vi "DAQ 1SDI v6.1.vi"() -> ()   [LabVIEW 2013]
uses:
  Strict Type Defs/type_meas_enum.ctl
  <instrlib>/niScope/Controls/niScope vertical coupling.ctl
panel:
  in  "stop":bool
  out "Loop count":i32=4690
  in  "Monitors":T1(tab)
  out "covariance HD 1 & 2":dbl(graph)=0.19831028169384832
  out "Conditional variance HD 1|2":dbl(graph)=1.0142124161365378
  out "Conditional variance HD 1|3":dbl(graph)=0.6065160666682574
  out "Conditional variance HD 2|3":dbl(graph)=0.5661489724627885
  out "covariance HD 1 & 3":dbl(graph)=-0.6559385878875881
  out "covariance HD 2 & 3":dbl(graph)=-0.6106758756892631
  in  "mode 2 polarity":bool
  out "Var(x1-x2/sqrt(2)-x3(sqrt(2))":dbl(graph)=0.19831028169384832
  out "Var(x2-x1/sqrt(2)-x3/sqrt(2))":dbl(graph)=-0.6559385878875881
  out "Var(x3-x1/sqrt(2)-x2/sqrt(2))":dbl(graph)=-0.6106758756892631
  in  "mode 3 polarity":bool
  in  "Settings":enum32{"Settings and Record", "Under the hood"}(tab)=enum."Under the hood"
  in  "Delay timing (ms)":u32(knob)=43 scale=0.0..250.0
  in  "Number of monitor samples":i32=10000 format="%.0p"
  in  "File location":path=path "C:/ni-rt/LabVIEW Data/July1/35dB109"
  in  "Type of measurement":T2=enum."electronic"
  in  "File root name":string="Real"
  in  "Number of samples save":i32=2000000 format="%.0p"
  in  "reset sn":bool
  in  "Shot noise start":bool
  in  "Additional text":string="OPA 1 optical power set to 15mV on HD A.\nOPA 2 optical power set to 15mV on HD B.\nLocal oscillator is set to 5V on HD.\nParametric gain set to 15 for OPA 1.\nParametric gain set to 15 for OPA 2.\nVertical range set to 0.5V for both channels.\nSample rate set to 14MS/s.\nMax input freq set to7MHz.\nVisibility between OPA 1 & OPA 2 = 99.6\nVisibility between OPA 1 & L.O.B = 98.9\nVisibility between OPA 1 & L.O. A = 98.9\nBoth squeezers expected to produce -7dB/11dB.\nLoss on EPR B =55.33% (3.5dB) \n"
  in  "Record":bool
  in  "Number of Files":i32=2
  out "File count":i32=1
  in  "Run":string="9"
  out "Cluster":T3={"Actual samples acquired ch 1"=120000, "Actual samples acquired ch 0"=120000, "Actual samples acquired ch 2"=120000}
  in  "Channel Parms":T5={"Input impedance (Ohms)"=2, "Maximum input frequency (Hz)"=7.0, "vertical coupling"=1, "Probe attenuation"=1.0, "Vertical range (V)"=1.0, "Vertical offset"=0.0, "channel enabled"=TRUE} {"Input impedance (Ohms)" items=["1 mega ohm"=0, "50 ohms"=2]; "Maximum input frequency (Hz)" format="%#_6p"; "vertical coupling" items=["AC", "DC", "Ground"]}
  in  "IIR filter specifications":T6={"Topology"=enum."Butterworth", "Type"=enum."Bandpass", "Order"=6, "Lower Fc"=2900000.0, "Upper Fc"=3100000.0, "PB Ripple"=1.0, "SB Attenuation"=60.0} {"PB Ripple" format="%0.2f"; "SB Attenuation" format="%0.2f"; "Lower Fc" format="%0.2p"; "Upper Fc" format="%0.2p"}
  out "error out":errorcluster caption="error out final"
  in  "max time (s)":dbl=10.0 caption="Time to run (s)"
  in  "Reference position":dbl(slide)=50.0 scale=0.0..100.0
  in  "Minimum sample rate (S/s)":dbl=14000000.0 format="%#_6p"
  out "Video bandwidth (Hz)":dbl=7.0
  in  "DAQ Cards":T7={"DAQ Card 1"="Dev2", "DAQ Card 2"="Dev3"}
  # "+1"
  # "-1"
  # "+1"
  # "-1"
  # "Variance won't be displayed until shot noise is taken"
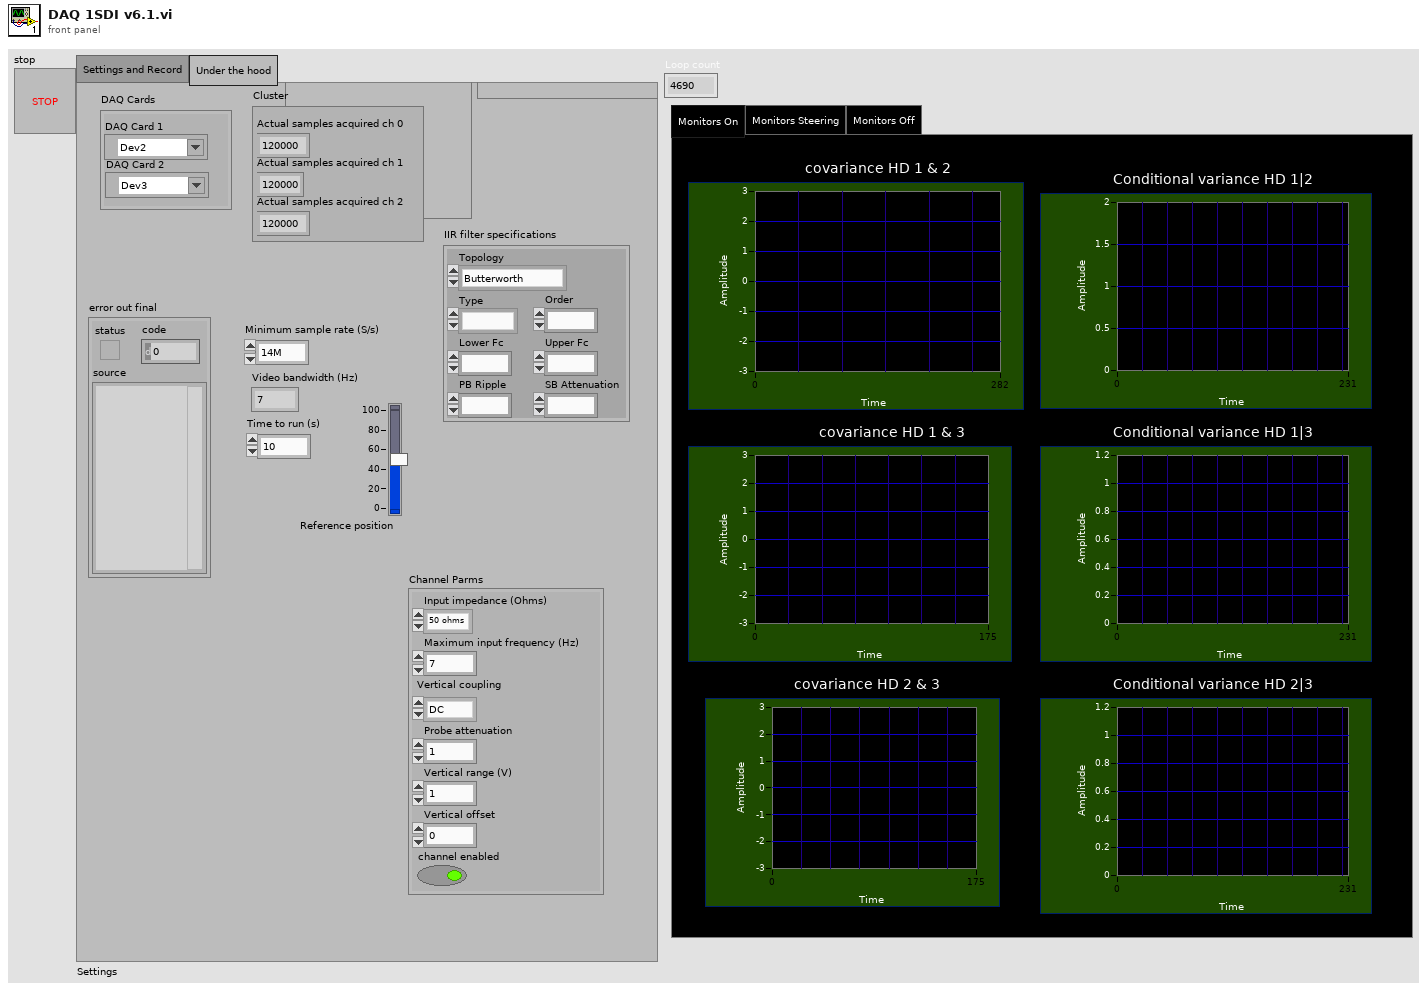
[diagram p1: front panel]
types:
  T1 = enum32{"Monitors On", "Monitors Steering", "Monitors Off"}
  T2 = typedef "type_meas_enum.ctl" = enum16{"shot", "x", "p", "electronic"}
  T3 = cluster{"Actual samples acquired ch 1":i32, "Actual samples acquired ch 0":i32, "Actual samples acquired ch 2":i32}
  T4 = typedef "niScope vertical coupling.ctl" = i32
  T5 = cluster{"Input impedance (Ohms)":u32, "Maximum input frequency (Hz)":dbl, "vertical coupling":T4, "Probe attenuation":dbl, "Vertical range (V)":dbl, "Vertical offset":dbl, "channel enabled":bool}
  T6 = cluster{"Topology":enum16{"Off", "Butterworth", "Chebyshev", "Inverse Chebyshev", "Elliptic", "Bessel"}, "Type":enum16{"Lowpass", "Highpass", "Bandpass", "Bandstop"}, "Order":i32, "Lower Fc":dbl, "Upper Fc":dbl, "PB Ripple":dbl, "SB Attenuation":dbl}
  T7 = cluster{"DAQ Card 1":refnum<k15>, "DAQ Card 2":refnum<k15>}
  T8 = cluster{"instrument handle":refnum<k15>, "instrument handle":refnum<k15>}
  T9 = cluster{"instrument handle out 0":refnum<k15>, "instrument handle out 1":refnum<k15>}
  T10 = cluster{"actualSamples":i32, "actualSamples":i32, "actualSamples":i32}
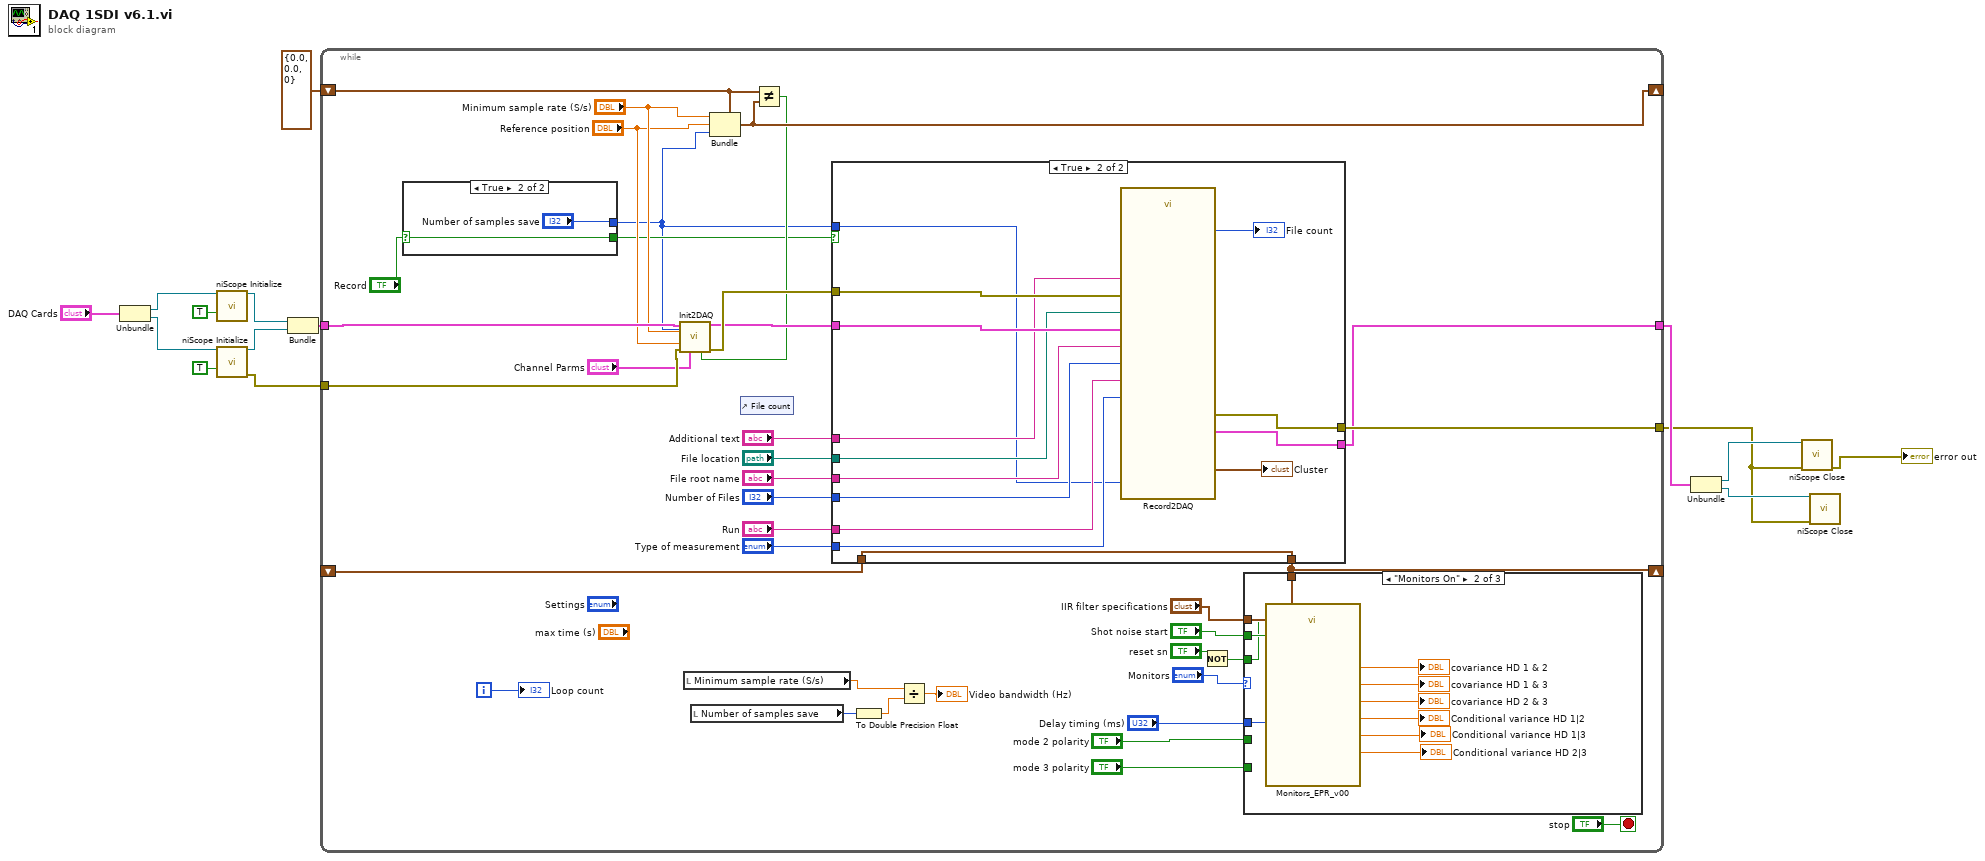
[diagram p0: block diagram]
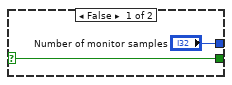
[diagram p2: hidden frame]
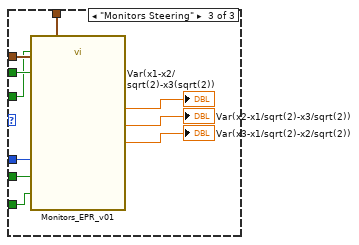
[diagram p4: hidden frame]
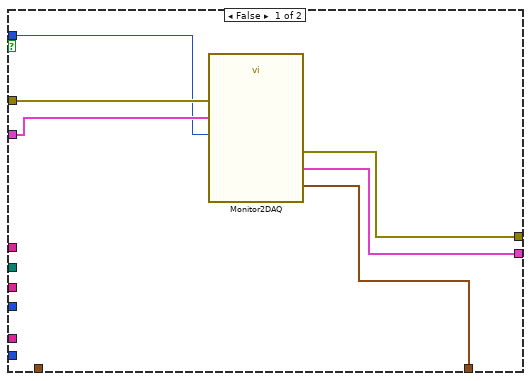
[diagram p5: hidden frame]
diagram:
  n1 = Unbundle("DAQ Cards") -> ("DAQ Card 1"=w7:refnum<k15>, "DAQ Card 2"=w6:refnum<k15>)
  n2 = call <instrlib>:"niScope Initialize.vi"("resource name"=w7, "reset device"=TRUE) -> ("instrument handle"=w4:refnum<k15>)  [unwired: 12 in, 1 out]
  n3 = call <instrlib>:"niScope Initialize.vi"("resource name"=w6, "reset device"=TRUE) -> ("instrument handle"=w3:refnum<k15>, "error out"=w5:errorcluster)  [unwired: 12 in]
  n4 = Bundle("instrument handle"=w4, "instrument handle"=w3) -> (w2:T8)  [unwired: 1 in]
  n5 = while {
    tunnel: [w46] -> w11
    tunnel: w5 -> [w32]
    shift-right: [w27] -> _
    shift-left: cluster{dbl, dbl, i32} {0.0, 0.0, 0} -> [w28]
    shift-right: [w22] -> _
    shift-left: _ -> [w21]
    tunnel: w2 -> [w33]
    tunnel: [w35] -> w15
    i -> [w48]
    stop <- "stop" stop-if-true
    n6 = case shown="True" "Record" {
      selector: "Record" -> [w54 w56]
      tunnel: ["Number of monitor samples" "Number of samples save"] -> w18
      tunnel: [w54 w56] -> w23
      frame False {
      }
      frame True {
      }
    }
    n7 = local read "Minimum sample rate (S/s)"() -> (w36:dbl)
    n8 = local read "Number of samples save"() -> (w38:i32)
    n9 = Bundle(cluster=w28, "Minimum sample rate (S/s)", "Reference position", w18) -> (w27:cluster{dbl, dbl, i32})
    n10 = control-ref of="File count"() -> ()  [unwired: 1 out]
    n11 = Not Equal?(x=w28, y=w27) -> (x != y?=w26:bool)
    n12 = call "Init2DAQ.vi"("resource names"=w33, "min record length"=w18, "min sample rate"="Minimum sample rate (S/s)", "reference position"="Reference position", "error in"=w32, "channel parms"="Channel Parms", "Ch param"=w26) -> ("instrument out"=w34:T9, "error out"=w52:errorcluster)  [unwired: 7 in]
    n13 = case shown="True" w23 {
      tunnel: w34 -> [w82 w97]
      tunnel: w52 -> [w83 w96]
      tunnel: [w81 w95] -> w46
      tunnel: "Additional text" -> [_ w94]
      tunnel: "File location" -> [_ w93]
      tunnel: "File root name" -> [_ w92]
      tunnel: "Number of Files" -> [_ w91]
      tunnel: "Run" -> [_ w90]
      tunnel: "Type of measurement" -> [_ w89]
      tunnel: [w80 w85] -> w22
      tunnel: [w79 w86] -> w35
      tunnel: w21 -> [_ w85]
      tunnel: w18 -> [w78 w84]
      frame False {
        n14 = call "Monitor2DAQ.vi"("instrument in"=w82, "error in"=w83, "numSamples"=w78) -> ("instrument out"=w79:T9, "wfm"=w80:waveform(dbl)[], "error out"=w81:errorcluster)  [unwired: 10 in]
      }
      frame True {
        n15 = call "Record2DAQ.vi"("instrument in"=w97, "Additional text"=w94, "numSamples"=w84, "File location"=w93, "Type of\nmeasurement"=w89, "Name root"=w92, "error in"=w96, "Run"=w90, "number of files"=w91) -> ("output cluster"=→"Cluster":T10, "instrument out"=w86:T9, "File count"=→"File count":i32, "error out"=w95:errorcluster)  [unwired: 2 in, 1 out]
      }
    }
    n16 = To Double Precision Float(number=w38) -> (double precision float=w37:dbl)
    n17 = Divide(x=w36, y=w37) -> (x/y=→"Video bandwidth (Hz)":dbl)
    n18 = Not(x="reset sn") -> (.not. x?=w31:bool)
    n19 = case shown="\"Monitors On\"" "Monitors" {
      tunnel: "Shot noise start" -> [_ w67 w77]
      tunnel: "IIR filter specifications" -> [_ w66 w76]
      tunnel: w31 -> [_ w65 w75]
      tunnel: w22 -> [_ w64 w74]
      tunnel: "Delay timing (ms)" -> [_ w57 w70]
      tunnel: "mode 2 polarity" -> [_ _ w69]
      tunnel: "mode 3 polarity" -> [_ _ w68]
      frame "Monitors Off" {
      }
      frame "Monitors On" {
        n20 = call "Monitors_EPR_v00.vi"("IIR filter specifications"=w66, "Wait(mSec)"=w57, "reset SN"=w65, "Shot noise start"=w67, "wfm"=w64) -> ("covariance B01"=→"covariance HD 1 & 2":dbl, "covariance B0A"=→"covariance HD 1 & 3":dbl, "covariance B1A"=→"covariance HD 2 & 3":dbl, "conditional variance B0|1"=→"Conditional variance HD 1|2":dbl, "conditional variance B1|A"=→"Conditional variance HD 2|3":dbl, "conditional variance B0|A"=→"Conditional variance HD 1|3":dbl)  [unwired: 5 in]
      }
      frame "Monitors Steering" {
        n21 = call "Monitors_EPR_v01.vi"("IIR filter specifications"=w76, "Wait(mSec)"=w70, "reset SN"=w75, "mode 2 polarity(T=+ve)"=w69, "Shot noise start"=w77, "wfm"=w74, "mode 3 polarity(T=+ve)"=w68) -> ("Var(x1-x2/sqrt(2)-x3/sqrt(2))"=→"Var(x1-x2/sqrt(2)-x3(sqrt(2))":dbl, "Var(x2-x1/sqrt(2)-x3/sqrt(2))"=→"Var(x2-x1/sqrt(2)-x3/sqrt(2))":dbl, "Var(x3-x1/sqrt(2)-x2/sqrt(2))"=→"Var(x3-x1/sqrt(2)-x2/sqrt(2))":dbl)  [unwired: 6 in]
      }
    }
    "Loop count" <- w48
  }
  n22 = Unbundle(w15) -> ("instrument handle out 0"=w14:refnum<k15>, "instrument handle out 1"=w13:refnum<k15>)
  n23 = call <instrlib>:"niScope Close.vi"("instrument handle"=w14, "error in"=w11) -> ("error out"=→"error out":errorcluster)  [unwired: 13 in]
  n24 = call <instrlib>:"niScope Close.vi"("instrument handle"=w13, "error in"=w11) -> ()  [unwired: 13 in, 1 out]
